vi "Library - Memory.vi"(7 "Msg Chain":string, 8 "error in (no error)":errorcluster {"code" format="Error %.0f"}, 10 "Libraries":refnum<class "Library Documentation.lvclass">[](array[class]), 11 "VIDoc Printer In":refnum<class "VIDoc Printer.lvclass">) -> (0 "error out":errorcluster {"code" format="Error %.0f"}, 3 "VIDoc Printer Out":refnum<class "VIDoc Printer.lvclass">)   [LabVIEW 2023, in "VIDoc Printer.lvlib" / "VIDoc Printer.lvclass"]
uses:
  VIDoc Printer.lvclass
  Parsing/Library Documentation/Library Documentation.lvclass
  VIDoc Printer.lvclass/VIDoc Printer.ctl
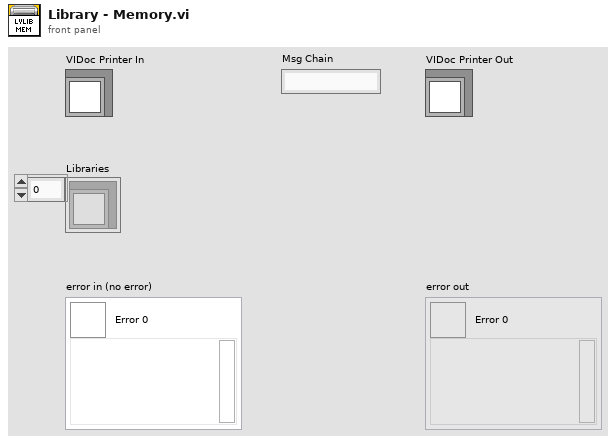
[diagram p1: front panel]
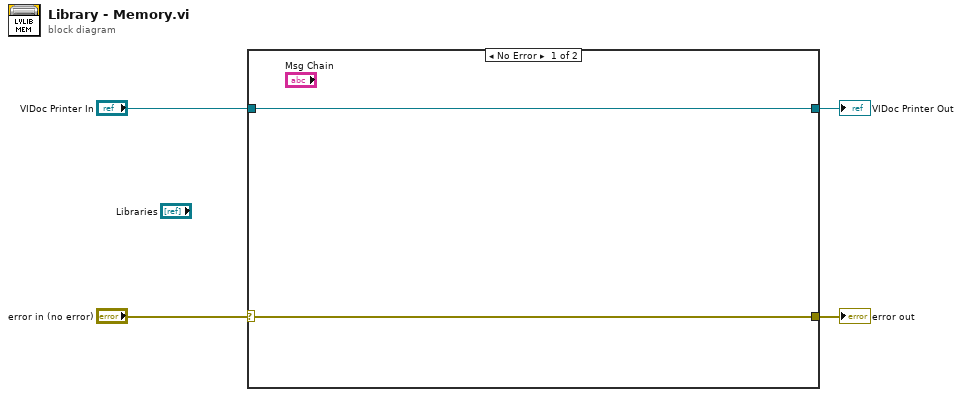
[diagram p0: block diagram]
diagram:
  n1 = case shown="No Error" "error in (no error)" {
    selector: "error in (no error)" -> [w5 w8]
    tunnel: [w5 w8] -> w3
    tunnel: [w6 w7] -> w1
    tunnel: "VIDoc Printer In" -> [w6 w7]
    frame No Error {
    }
    frame Error {
    }
  }
  "error out" <- w3
  "VIDoc Printer Out" <- w1
